vi "readU32FIFO.vi"(8 "error in (no error)":errorcluster, 9 "Timeout":i32, 10 "NumberOfElements":u32, 11 "HealthAndStatusDataFIFO in":refnum<class "HealthAndStatusDataFIFO.lvclass">) -> (0 "error out":errorcluster, 1 "ElementsRemaining":u32, 2 "Data":u32[](array[numeric]), 3 "HealthAndStatusDataFIFO out":refnum<class "HealthAndStatusDataFIFO.lvclass">)   [LabVIEW 2016, in "HealthAndStatusDataFIFO.lvclass"]
uses:
  HealthAndStatusDataFIFO.lvclass
  HealthAndStatusDataFIFO.lvclass/HealthAndStatusDataFIFO.ctl
  FPGA/FPGA.lvclass
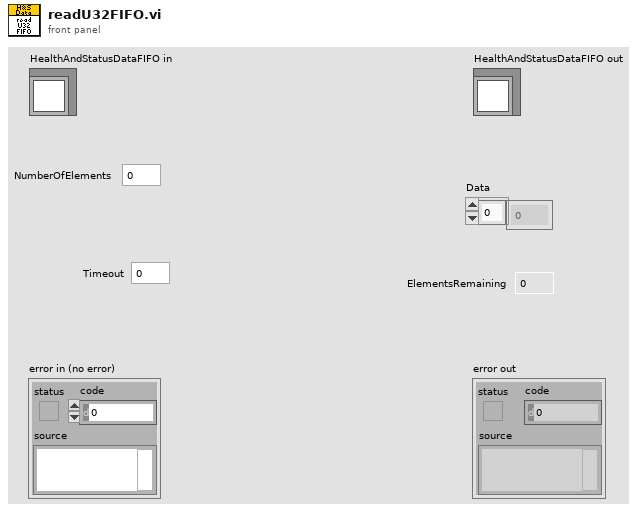
[diagram p1: front panel]
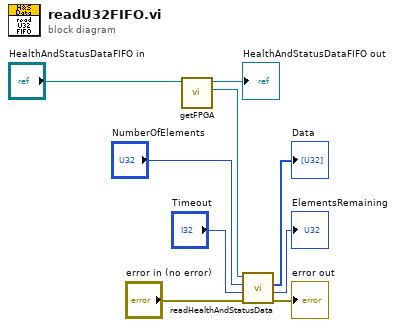
[diagram p0: block diagram]
diagram:
  n1 = call "getFPGA.vi"("HealthAndStatusDataFIFO in"="HealthAndStatusDataFIFO in") -> ("FPGA"=w7:refnum<class "FPGA.lvclass">, "HealthAndStatusDataFIFO out"=→"HealthAndStatusDataFIFO out":refnum<class "HealthAndStatusDataFIFO.lvclass">)  [unwired: 9 in]
  n2 = call "readHealthAndStatusData.vi"("error in (no error)"="error in (no error)", "Timeout"="Timeout", "NumberOfElements"="NumberOfElements", "FPGA in"=w7) -> ("error out"=→"error out":errorcluster, "ElementsRemaining"=→"ElementsRemaining":u32, "Data"=→"Data":u32[])  [unwired: 4 in, 1 out]
